vi "task.ongoing_lua.vi"(5 "LuaVIEW reference":T1) -> (15 "error out":errorcluster)   [LabVIEW 2012]
doc: "Tests if a task is ongoing. A started task is ongoing until it has run to completion (of the task script), suffers and error, is stopped, or is killed. This implies that tasks that are initializing, running, or paused are all ongoing.\nParameters:\nstr:task_identifier\nResults:\nbool:ongoing"
uses:
  typedefs/t_LuaVIEW Reference.ctl
  typedefs/t_LuaVIEW Task List Methods.ctl
  subvis/private/LuaVIEW Pull (string).vi
  subvis/private/LuaVIEW Push (boolean).vi
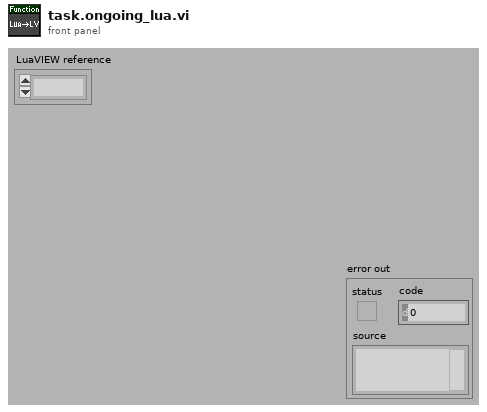
[diagram p1: front panel]
types:
  T1 = typedef "t_LuaVIEW Reference.ctl" = refnum<k1>
  T2 = typedef "t_LuaVIEW Task List Methods.ctl" = enum16{"clear list", "add", "test", "remove", "get ref", "get task info", "get list", "get script info", "ongoing?", "resume", "pause", "stop", "confirm", "message"}
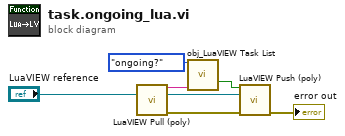
[diagram p0: block diagram]
diagram:
  n1 = call-poly "LuaVIEW Pull (poly).vi"("LuaVIEW reference in"="LuaVIEW reference") -> ("string"=w3:string, "LuaVIEW reference out"=w4:T1, "error out"=w2:errorcluster)  [unwired: 12 in]
  n2 = call "obj_LuaVIEW Task List.vi"("method"=t_LuaVIEW_Task_List_Methods."ongoing?", "task identifier"=w3) -> ("set/ongoing"=w7:bool)  [unwired: 8 in, 5 out]
  n3 = call-poly "LuaVIEW Push (poly).vi"("boolean"=w7, "LuaVIEW reference in"=w4, "error in (no error)"=w2) -> ("error out"=→"error out":errorcluster)  [unwired: 11 in, 1 out]
